vi "UHR-Fleezers Control (host) -TL FB Corrected Ronen semipassive.vi"(0 "Tab Control":T5(tab)=enum."Trap Control (RF)") -> ()   [LabVIEW 2013] (continued)
        n1854 = Array Subset(array=w2700, index (col)=w2689) -> (w2697:dbl[][])  [unwired: 3 in]
        n1855 = Array Subset(array=w2774, index (col)=0 ("index"), length (col)=w2689) -> (w2773:dbl[][])  [unwired: 2 in]
        n1856 = Array Subset(array=w2774, index (col)=w2689) -> (w2771:dbl[][])  [unwired: 3 in]
        n1857 = Array Subset(array=w2757, index (col)=0 ("index"), length (col)=w2689) -> (w2762:dbl[][])  [unwired: 2 in]
        n1858 = Array Subset(array=w2757, index (col)=w2689) -> (w2760:dbl[][])  [unwired: 3 in]
        n1859 = for {
          tunnel: w2769 -> [w2811] mode=indexing
          tunnel: [w2810] -> w2768 mode=indexing
          workers-P: _ -> [_]
          n1860 = Reverse 1D Array(array=w2811) -> (reversed array=w2810:dbl[])
        }
        n1861 = for {
          tunnel: w2755 -> [w2807] mode=indexing
          tunnel: [w2806] -> w2754 mode=indexing
          workers-P: _ -> [_]
          n1862 = Reverse 1D Array(array=w2807) -> (reversed array=w2806:dbl[])
        }
        n1863 = for {
          tunnel: w2699 -> [w2805] mode=indexing
          tunnel: [w2804] -> w2698 mode=indexing
          workers-P: _ -> [_]
          n1864 = Reverse 1D Array(array=w2805) -> (reversed array=w2804:dbl[])
        }
        n1865 = for {
          tunnel: w2773 -> [w2813] mode=indexing
          tunnel: [w2812] -> w2772 mode=indexing
          workers-P: _ -> [_]
          n1866 = Reverse 1D Array(array=w2813) -> (reversed array=w2812:dbl[])
        }
        n1867 = for {
          tunnel: w2762 -> [w2809] mode=indexing
          tunnel: [w2808] -> w2761 mode=indexing
          workers-P: _ -> [_]
          n1868 = Reverse 1D Array(array=w2809) -> (reversed array=w2808:dbl[])
        }
        n1869 = Index Array(array=w2774, index (row)=0) -> (element=→"Waveform Graph":dbl[])  [unwired: 1 in]
        n1870 = Add(x=w2768, y=w2767) -> (x+y=w2766:dbl[][])
        n1871 = Add(x=w2754, y=w2753) -> (x+y=w2752:dbl[][])
        n1872 = Add(x=w2698, y=w2697) -> (x+y=w2682:dbl[][])
        n1873 = Add(x=w2772, y=w2771) -> (x+y=w2746:dbl[][])
        n1874 = Add(x=w2761, y=w2760) -> (x+y=w2759:dbl[][])
        n1875 = Divide(x=w2752, y=2) -> (x/y=w2750:dbl[][])
        n1876 = Divide(x=w2766, y=2) -> (x/y=w2711:dbl[][])
        n1877 = Divide(x=w2759, y=2) -> (x/y=w2713:dbl[][])
        n1878 = To Single Precision Float(number=w2746) -> (single precision float=w2745:sgl[][])
        n1879 = Transpose 2D Array(2D array=w2750) -> (transposed array=→"Data map":dbl[][])
        n1880 = To Single Precision Float(number=w2682) -> (single precision float=w2686:sgl[][])
        n1881 = To Single Precision Float(number=w2711) -> (single precision float=w2717:sgl[][])
        n1882 = To Single Precision Float(number=w2713) -> (single precision float=w2714:sgl[][])
        n1883 = call "IMAQ ArrayToImage"("Image Pixels (Float)"=w2745, "Image"=w2679) -> ("Image Out"=w2748:T3)  [unwired: 8 in, 1 out]
        n1884 = call "IMAQ ArrayToImage"("Image Pixels (Float)"=w2686, "Image"=w2678) -> ("Image Out"=w2688:T3)  [unwired: 8 in, 1 out]
        n1885 = call "IMAQ ArrayToImage"("Image Pixels (Float)"=w2717, "Image"=w2677) -> ("Image Out"=w2719:T3)  [unwired: 8 in, 1 out]
        n1886 = call "IMAQ ArrayToImage"("Image Pixels (Float)"=w2714, "Image"=w2676) -> ("Image Out"=w2716:T3)  [unwired: 8 in, 1 out]
        n1887 = call "IMAQ Symmetry"("Type of Symmetry"=w2747, "Image Src"=w2748) -> ("Image Dst Out"=w2743:T3)  [unwired: 3 in, 1 out]
        n1888 = call "IMAQ Symmetry"("Type of Symmetry"=w2687, "Image Src"=w2688) -> ("Image Dst Out"=w2684:T3)  [unwired: 3 in, 1 out]
        n1889 = call "IMAQ Symmetry"("Type of Symmetry"=w2718, "Image Src"=w2719) -> ("Image Dst Out"=→"Detection Laser X":T3)  [unwired: 3 in, 1 out]
        n1890 = call "IMAQ Symmetry"("Type of Symmetry"=w2715, "Image Src"=w2716) -> ("Image Dst Out"=→"Detection Laser Y":T3)  [unwired: 3 in, 1 out]
        n1891 = call "IMAQ Set Simple Calibration"("Calibration Axis Info"=T37 {"Origin Pixel"={"X"=0.0, "Y"=0.0}, "Angle Relative to Horizontal (deg)"=0.0, "Axis Reference"=0}, "Grid Descriptor"=T38 {"X Step"=0.3, "Y Step"=0.3, "Unit"=enum."Undefined"}, "Image"=w2743) -> ("Calibrated Image"=→"APD 1":T3)  [unwired: 7 in, 1 out]
        n1892 = call "IMAQ Set Simple Calibration"("Calibration Axis Info"=T37 {"Origin Pixel"={"X"=0.0, "Y"=0.0}, "Angle Relative to Horizontal (deg)"=0.0, "Axis Reference"=0}, "Grid Descriptor"=T38 {"X Step"=0.3, "Y Step"=0.3, "Unit"=enum."Undefined"}, "Image"=w2684) -> ("Calibrated Image"=→"APD 2":T3)  [unwired: 7 in, 1 out]
      }
    }
    n1893 = Subtract(x=w2226, y="APD 2 Offset") -> (x-y=w2223:waveform(dbl))
    n1894 = Subtract(x=w2228, y="APD 1 Offset") -> (x-y=w2224:waveform(dbl))
    n1895 = Index Array(array=w2243, index=3) -> (element=w2310:waveform(dbl))
    n1896 = Index Array(array=w2243, index=6) -> (element=w2307:waveform(dbl))
    n1897 = Build Array(w2224, w2223) -> (→"APD Chart":waveform(dbl)[])
    n1898 = Array Size(array=w2300) -> (size(s)=w2350:i32)
    n1899 = call <vilib>:"Std Deviation and Variance.vi"("X"=w2236) -> ("standard deviation"=w2235:dbl)  [unwired: 1 in, 2 out]
    n1900 = Add Array Elements(numeric array=w2236) -> (sum=w2238:u32)
    n1901 = Add Array Elements(numeric array=w2300) -> (sum=w2360:u32)
    n1902 = call <vilib>:"Std Deviation and Variance.vi"("X"=w2300) -> ("standard deviation"=w2299:dbl)  [unwired: 1 in, 2 out]
    n1903 = Divide(x=w2235, y=w2234) -> (x/y=w2231:dbl)
    "Rate sigma (Hz) 2" <- w2231
    n1904 = Multiply(x=w2234, y=w2350) -> (x*y=w2237:dbl)
    "Int. Time (s)" <- w2237
    n1905 = Divide(x=w2238, y=w2237) -> (x/y=w2232:dbl)
    "APD 2 Rate (Hz)" <- w2232
    n1906 = Divide(x=w2360, y=w2237) -> (x/y=w2297:dbl)
    "APD 1 Rate (Hz)" <- w2297
    n1907 = Divide(x=w2299, y=w2234) -> (x/y=w2298:dbl)
    "Rate sigma (Hz)" <- w2298
    n1908 = Divide(x=w2231, y=w2232) -> (x/y=→"Sigma/Mean 2":dbl)
    n1909 = Divide(x=w2298, y=w2297) -> (x/y=→"Sigma/Mean":dbl)
    n1910 = case shown="2" "Calibration" {
      tunnel: "T1 alpha_x (nm/V)" -> [_ w2642 w2663]
      tunnel: "T1 kappa_x (pN/nm)" -> [_ _ w2653]
      tunnel: "T2 alpha_x (nm/V)" -> [_ w2641 w2661]
      tunnel: "T2 kappa_x (pN/nm)" -> [_ _ w2654]
      tunnel: w2310 -> [w2624 w2639 w2659]
      tunnel: w2307 -> [w2623 w2637 w2657]
      tunnel: [w2624 w2636 w2656] -> w2336
      tunnel: [w2623 w2635 w2655] -> w2335
      tunnel: ["T1 X (V)" ("Label.Text") "T1 X (nm)" ("Label.Text") "T1 X (pN)" ("Label.Text")] -> w2328
      tunnel: ["T2 X (V)" ("Label.Text") "T2 X (nm)" ("Label.Text") "T2 X (pN)" ("Label.Text")] -> w2327
      tunnel: ["Position (V)" ("Label.Text") "Position (nm)" ("Label.Text") "Force (pN)" ("Label.Text")] -> w2329
      tunnel: w2309 -> [_ w2627 w2646]
      tunnel: w2311 -> [_ w2630 w2648]
      tunnel: ["Mean (V)" ("Label.Text") "Mean (nm)" ("Label.Text") "Mean (pN)" ("Label.Text")] -> w2324
      tunnel: ["Difference (V)" ("Label.Text") "Difference (nm)" ("Label.Text") "Difference (pN)" ("Label.Text")] -> w2251
      frame 0, Default {
      }
      frame 1 {
        # "position"
        n1911 = Unbundle By Name(w2639) -> ("Y"=w2643:dbl[])
        n1912 = Unbundle By Name(w2637) -> ("Y"=w2628:dbl[])
        n1913 = Subtract(x=w2643, y=w2630) -> (x-y=w2631:dbl[])
        n1914 = Subtract(x=w2628, y=w2627) -> (x-y=w2629:dbl[])
        n1915 = Multiply(x=w2629, y=w2641) -> (x*y=w2638:dbl[])
        n1916 = Multiply(x=w2642, y=w2631) -> (x*y=w2640:dbl[])
        n1917 = Bundle By Name(cluster=w2637, "Y"=w2638) -> (w2635:waveform(dbl))
        n1918 = Bundle By Name(cluster=w2639, "Y"=w2640) -> (w2636:waveform(dbl))
      }
      frame 2 {
        # "force"
        n1919 = Unbundle By Name(w2659) -> ("Y"=w2664:dbl[])
        n1920 = Unbundle By Name(w2657) -> ("Y"=w2662:dbl[])
        n1921 = Subtract(x=w2662, y=w2646) -> (x-y=w2647:dbl[])
        n1922 = Subtract(x=w2664, y=w2648) -> (x-y=w2649:dbl[])
        n1923 = Compound Arithmetic op=MULTIPLY(w2647, w2661, w2654) -> (w2658:dbl[])
        n1924 = Compound Arithmetic op=MULTIPLY(w2653, w2663, w2649) -> (w2660:dbl[])
        n1925 = Bundle By Name(cluster=w2657, "Y"=w2658) -> (w2655:waveform(dbl))
        n1926 = Bundle By Name(cluster=w2659, "Y"=w2660) -> (w2656:waveform(dbl))
      }
    }
    n1927 = feedback-in #17("Calibration") -> ()
    n1928 = feedback #17(u16 1 ("Calibration")) -> (w2331:u16)
    n1929 = local read "Trap 2 Bead Size (nm)"() -> (w2131:dbl)
    n1930 = local read "Trap 1 Bead Size (nm)"() -> (w2130:dbl)
    n1931 = local read "AOM X Cal (nm/MHz)"() -> (w2128:dbl)
    n1932 = local read "Trap Delta (MHz)"() -> (w2127:dbl)
    n1933 = Not Equal?(x=w2331, y="Calibration") -> (x != y?=w2288:bool)
    n1934 = Multiply(x=w2128, y=w2127) -> (x*y=w2132:dbl)
    n1935 = Add(x=w2131, y=w2130) -> (x+y=w2134:dbl)
    n1936 = Unbundle By Name(w2310) -> ("Y"=w2313:dbl[])
    n1937 = Unbundle By Name(w2307) -> ("Y"=w2316:dbl[])
    n1938 = Divide(x=w2134, y=2.0) -> (x/y=w2129:dbl)
    n1939 = Subtract(x=w2313, y=w2311) -> (x-y=w2314:dbl[])
    n1940 = Subtract(x=w2316, y=w2309) -> (x-y=w2315:dbl[])
    n1941 = disable-structure shown="Enabled" {
      disable-tunnel: [-1.0 ("y") 1.0] -> w2317
      frame Disabled {
      }
      frame Enabled {
      }
    }
    n1942 = Multiply(x=w2315, y="T2 alpha_x (nm/V)") -> (x*y=w2306:dbl[])
    n1943 = Multiply(x="T1 alpha_x (nm/V)", y=w2314) -> (x*y=w2305:dbl[])
    n1944 = Multiply(x=w2335, y=w2317) -> (x*y=w2318:waveform(dbl))
    n1945 = case shown="False" "Read Lateness and Rel Phase" {
      tunnel: w2104 -> [w2590 w2612]
      tunnel: w2143 -> [w2591 w2611]
      tunnel: [w2590 w2610] -> w2303
      tunnel: [w2591 w2609] -> w2302
      frame False {
      }
      frame True {
        n1946 = xnode "Read/Write Control"("FPGA VI Reference In"=w2612, "error in"=w2611) -> ("FPGA VI Reference Out"=w2610:T20, "error out"=w2609:errorcluster, "GI Relative phase"=→"GI relative phase":i16, "Relative phase"=→"Relative phase (AI1)":i16, "AI Late Counter"=→"Late Counter (AI1)":u16, "GI Late Counter"=→"GI Late Counter":u16, "MCL Late Counter"=→"MCL Late Counter":u16, "MCL Relative Phase"=→"Relative Phase (MCL)":i16, "APD Acq Relative Phase"=→"APD Acq Relative Phase":i16, "APD 1 Gate Relative Phase"=→"APD 1 Gate Relative Phase":i16, "APD 2 Gate Relative Phase"=→"APD 2 Gate Relative Phase":i16, "APD Acq Late Counter"=→"APD Acq Late Counter":u16, "APD 1 Gate Late Counter"=→"APD 1 Gate Late Counter":u16, "APD 2 Gate Late Counter"=→"APD 2 Gate Late Counter":u16, "Green FB Relative Phase"=→"Relative phase (Green FB)":i16, "GI Relative phase 2"=→"GI relative phase 2":i16, "GI Late Counter 2"=→"GI Late Counter 2":u16, "Trap Pos FIFO Timeout"=→"Trap Pos FIFO Timeout":u16, "Trap AI FIFO Timeout"=→"Trap AI FIFO Timeout":u16)
      }
    }
    n1947 = Subtract(x=w2306, y=w2305) -> (x-y=w2126:dbl[])
    n1948 = call-poly <vilib>:"Mean.vi"("X"=w2126) -> ("mean"=w2133:dbl)  [unwired: 1 out]
    n1949 = Add(x=w2132, y=w2133) -> (x+y=w2136:dbl)
    n1950 = Subtract(x=w2136, y=w2129) -> (x-y=→"Tether Extension (nm, calculated)":dbl)
    n1951 = Unbundle By Name(w2335) -> ("Y"=w2276:dbl[])
    n1952 = Unbundle By Name(w2336) -> ("Y"=w2277:dbl[])
    n1953 = Build Array(w2336, w2318) -> (→"Force":waveform(dbl)[])
    n1954 = Subtract(x=w2126, y="Offset (nm)") -> (x-y=w2274:dbl[])
    n1955 = call-poly <vilib>:"Mean.vi"("X"=w2276) -> ("mean"=w2255:dbl)  [unwired: 1 out]
    "T2 X" <- w2255
    n1956 = Absolute Value(x=w2277) -> (abs(x)=w2278:dbl[])
    n1957 = Absolute Value(x=w2276) -> (abs(x)=w2279:dbl[])
    n1958 = call-poly <vilib>:"Mean.vi"("X"=w2277) -> ("mean"=w2256:dbl)  [unwired: 1 out]
    "T1 X" <- w2256
    n1959 = Add(x=w2278, y=w2279) -> (x+y=w2280:dbl[])
    n1960 = Bundle By Name(cluster=w2310, "Y"=w2274) -> (w2242:waveform(dbl))
    "Bead Separation" <- w2242
    n1961 = Divide(x=w2280, y=2.0) -> (x/y=→"Vec Mean of T1 T2":dbl[])
    n1962 = case shown="True" w2288 {
      tunnel: w2329 -> [_ w2617]
      tunnel: w2328 -> [_ w2616]
      tunnel: w2327 -> [_ w2615]
      tunnel: w2324 -> [_ w2614]
      tunnel: w2251 -> [_ w2613]
      frame False {
      }
      frame True {
        n1963 = property on="Force" class="WFChart (strict)"("YScale.NameLbl.Text"=w2617) -> ()  [unwired: 2 in, 2 out]
        n1964 = property on="T2 X" class="DigNum (strict)"("Caption.Text"=w2615) -> ()  [unwired: 2 in, 2 out]
        n1965 = property on="T1 X" class="DigNum (strict)"("Caption.Text"=w2616) -> ()  [unwired: 2 in, 2 out]
        n1966 = property on="Mean" class="DigNum (strict)"("Caption.Text"=w2614) -> ()  [unwired: 2 in, 2 out]
        n1967 = property on="Difference" class="DigNum (strict)"("Caption.Text"=w2613) -> ()  [unwired: 2 in, 2 out]
      }
    }
    n1968 = local read "Tether"() -> (w2282:bool)
    n1969 = Absolute Value(x=w2256) -> (abs(x)=w2253:dbl)
    n1970 = Absolute Value(x=w2255) -> (abs(x)=w2252:dbl)
    n1971 = Add(x=w2253, y=w2252) -> (x+y=w2326:dbl)
    n1972 = Subtract(x=w2253, y=w2252) -> (x-y=→"Difference":dbl)
    n1973 = feedback #18(w2274) -> (w2273:dbl[])
    n1974 = Divide(x=w2326, y=2.0) -> (x/y=w2101:dbl)
    "Mean" <- w2101
    n1975 = case shown="True" w2282 {
      tunnel: w2101 -> [_ w2549]
      frame False {
      }
      frame True {
        n1976 = Greater?(x="Lost Tether Alarm Threshold (pN)", y=w2549) -> (0:w2547:bool)
        n1977 = case shown="True" w2547 {
          frame False {
          }
          frame True {
            n1978 = flat-sequence {
              frame #0 {
                # "stop only if saving"
                n1979 = local read "Saving..."() -> (w2562:bool)
                n1980 = And(x=w2562, y="TA Cancel Save?") -> (x .and. y?=w2561:bool)
                n1981 = local write "Stop Saving"(w2561) -> ()
              }
              frame #1 {
                n1982 = case shown="True" "TA Green Off?" {
                  frame False {
                  }
                  frame True {
                    w2565 = FALSE ("Fl. Triggered...")
                    n1983 = local write "Fl. Triggered..."(w2565) -> ()
                    n1984 = property on="Green Laser ON/Interlacing" class="Bool (strict)"("Val(Sgnl)"=w2565) -> ()  [unwired: 2 in, 2 out]
                  }
                }
              }
            }
            n1985 = local read "Time tether formed"() -> (w2556:timestamp)
            n1986 = Get Date/Time In Seconds() -> (seconds since 1Jan1904=w2557:timestamp)
            n1987 = Subtract(x=w2557, y=w2556) -> (x-y=w2555:dbl)
            n1988 = Number To Decimal String(number=w2555) -> (decimal integer string=w2552:string)  [unwired: 1 out]
            n1989 = local read "Messages"() -> (w2559:string)
            n1990 = call <vilib>:"Beep.vi"() -> ()  [unwired: 3 in, 9 out]
            n1991 = Concatenate Strings("Lost tether (" ("Message to add"), w2552, " s)." ("string")) -> (w2554:string)
            n1992 = local write "Tether"(FALSE ("Tether")) -> ()
            n1993 = call "Update messages.vi"("Message to add"=w2554, "Old message string"=w2559) -> ("New message string"=w2558:string)
            n1994 = local write "Messages"(w2558) -> ()
            n1995 = property on="Trap Pos. FB ON" class="Bool (strict)"("Val(Sgnl)"=FALSE ("Value (Signaling)")) -> ()  [unwired: 2 in, 2 out]
          }
        }
      }
    }
    n1996 = Build Array (concatenate)(w2274, w2273) -> (w2272:dbl[])
    n1997 = Split 1D Array(array=w2272, index=w2154) -> (first subarray=w2268:dbl[])  [unwired: 1 out]
    n1998 = feedback-in #18(w2268) -> ()
    n1999 = call-poly <vilib>:"Mean.vi"("X"=w2268) -> ("mean"=w2267:dbl)  [unwired: 1 out]
    "Bead Mean (nm)" <- w2267
    n2000 = Subtract(x=w2268, y=w2267) -> (x-y=w2266:dbl[])
    n2001 = Square(x=w2266) -> (x^2=w2265:dbl[])
    n2002 = case shown="True" "Semi Passive ON" {
      tunnel: "Semi Passive mode" -> [_ w2428]
      tunnel: "Jump Force (pN)" -> [_ w2427]
      tunnel: w2101 -> [_ w2426]
      frame False {
      }
      frame True {
        n2003 = case shown="\"Use Feedback\"" w2428 {
          tunnel: w2427 -> [_ w2431 w2447]
          tunnel: w2426 -> [_ w2430 w2446]
          frame "None" {
          }
          frame "Use Feedback" {
            n2004 = local read "Target Force (pN)"() -> (w2433:dbl)
            n2005 = Less?(x=w2431, y=w2433) -> (x < y?=w2432:bool)
            n2006 = case shown="True" w2432 {
              tunnel: w2431 -> [w2440 w2443]
              tunnel: w2430 -> [w2439 w2442]
              tunnel: [w2438 w2441] -> w2429
              frame False {
                n2007 = Less?(x=w2440, y=w2439) -> (x < y?=w2438:bool)
              }
              frame True {
                n2008 = Greater?(x=w2443, y=w2442) -> (0:w2441:bool)
              }
            }
            n2009 = case shown="True" w2429 {
              frame False {
                n2010 = local read "Trap Pos. FB ON"() -> (w2434:bool)
                n2011 = case shown="True" w2434 {
                  frame False {
                  }
                  frame True {
                    n2012 = property on="Trap Pos. FB ON" class="Bool (strict)"("Val(Sgnl)"=FALSE) -> ()  [unwired: 2 in, 2 out]
                  }
                }
              }
              frame True {
                n2013 = local read "Trap Pos. FB ON"() -> (w2436:bool)
                n2014 = case shown="False" w2436 {
                  frame False {
                    n2015 = property on="Trap Pos. FB ON" class="Bool (strict)"("Val(Sgnl)"=TRUE) -> ()  [unwired: 2 in, 2 out]
                  }
                  frame True {
                  }
                }
              }
            }
          }
          frame "Sharp Jump" {
            n2016 = local read "Target Force (pN)"() -> (w2449:dbl)
            n2017 = Greater?(x=w2447, y=w2449) -> (0:w2448:bool)
            n2018 = case shown="True" w2448 {
              tunnel: w2447 -> [w2464 w2468]
              tunnel: w2446 -> [w2465 w2467]
              tunnel: [w2463 w2466] -> w2445
              frame False {
                n2019 = Greater?(x=w2465, y=w2464) -> (0:w2463:bool)
              }
              frame True {
                n2020 = Less?(x=w2468, y=w2467) -> (x < y?=w2466:bool)
              }
            }
            n2021 = Subtract(x=w2447, y=w2449) -> (x-y=w2444:dbl)
            n2022 = case shown="True" w2445 {
              tunnel: w2444 -> [_ w2455]
              frame False {
              }
              frame True {
                n2023 = local read "T1 kappa_x (pN/nm)"() -> (w2460:dbl)
                n2024 = local read "T2 kappa_x (pN/nm)"() -> (w2461:dbl)
                n2025 = Reciprocal(x="DNA stiffness (pN / nm)") -> (1/x=w2457:dbl)
                n2026 = Reciprocal(x=w2460) -> (1/x=w2459:dbl)
                n2027 = Reciprocal(x=w2461) -> (1/x=w2458:dbl)
                n2028 = Compound Arithmetic op=ADD(w2459, w2458, w2457) -> (w2456:dbl)
                n2029 = local read "AOM X Cal (nm/MHz)"() -> (w2454:dbl)
                n2030 = Multiply(x=w2456, y=w2455) -> (x*y=w2453:dbl)
                n2031 = local read "Trap Delta (MHz)"() -> (w2451:dbl)
                n2032 = Divide(x=w2453, y=w2454) -> (x/y=w2452:dbl)
                n2033 = Subtract(x=w2451, y=w2452) -> (x-y=w2450:dbl)
                n2034 = property on="Trap Delta (MHz)" class="DigNum (strict)"("Val(Sgnl)"=w2450) -> ()  [unwired: 2 in, 2 out]
              }
            }
          }
        }
      }
    }
    n2035 = call-poly <vilib>:"Mean.vi"("X"=w2265) -> ("mean"=w2264:dbl)  [unwired: 1 out]
    n2036 = Square Root(x=w2264) -> (sqrt(x)=w2263:dbl)
    n2037 = Multiply(x=10.0, y=w2263) -> (x*y=→"RMS (Ang)":dbl)
    n2038 = xnode "Read/Write Control"("FPGA VI Reference In"=w2303, "error in"=w2302) -> ("FPGA VI Reference Out"=w2414:T20, "error out"=w2408:errorcluster, "AI4 Y Sum Set 1"=w2404:i16, "AI4 Y Sum Set 2"=w2403:i16, "AI1 X Set 1"=w2188:fxp<+/-,16,1>, "AI1 X Set 2"=w2187:fxp<+/-,16,1>, "Trap Pos FB Int Signal"=→"Trap Pos FB Int Signal":fxp<+/-,24,9>, "Trap Pos FB Int-Norm Signal"=→"Trap Pos FB Int-Norm Signal":fxp<+/-,24,9>, "Trap Pos FB Action"=w2181:i64, "Scanning"=→"AOD Scanning":bool, "Scan I"=→"AOD Scan I":u64, "Scanning MCL"=w2406:bool, "Scan I (MCL)"=→"MCL Scan I":u64, "Green FB Signals"=w2345:T48)  [unwired: 1 out]
    "MCL Scanning" <- w2406
    "Trap Pos FB Action" <- w2181
    n2039 = local read "AI2 (V)"() -> (w2405:cluster{"Set 1":dbl, "Set 2":dbl})
    n2040 = Bundle By Name(cluster=w2405, "Set 1"=w2404, "Set 2"=w2403) -> (w2401:cluster{"Set 1":dbl, "Set 2":dbl})
    n2041 = Divide(x=w2181, y=327.67) -> (x/y=→"Action (%)":dbl)
    n2042 = local read "Trap X (AI1)"() -> (w2201:T1)
    n2043 = Divide(x=w2401, y=3276.7) -> (x/y=w2400:cluster{"Set 1":dbl, "Set 2":dbl})
    n2044 = local write "AI2 (V)"(w2400) -> ()
    n2045 = Bundle(cluster=w2201, "Trap 1"=w2188, "Trap 2"=w2187) -> (→"Trap X (AI1)":T1)
    n2046 = Divide(x=w2345, y=3276.7) -> (x/y=w2341:T49)
    n2047 = Unbundle By Name(w2341) -> ("Green FB Ch 0"=w2344:dbl, "Green FB Ch 1"=w2343:dbl, "Green FB Ch 2"=w2342:dbl)
    n2048 = Divide(x=w2344, y=w2342) -> (x/y=w2340:dbl)
    n2049 = Divide(x=w2343, y=w2342) -> (x/y=w2339:dbl)
    n2050 = flat-sequence "To save data" {
      tunnel: [w3439] -> w2425
      tunnel: [w3440] -> w2424
      tunnel: w2376 -> [w3433]
      tunnel: w2270 -> [w3437]
      tunnel: ["Save Calibration"] -> w2397
      tunnel: w2394 -> [w3436]
      tunnel: [w3429] -> w2393
      tunnel: [w3426] -> w2392
      tunnel: [w3423] -> w2391
      tunnel: w2375 -> [w3425]
      tunnel: w2286 -> [w3419]
      tunnel: [w3419] -> w2285
      tunnel: ["Start Saving"] -> w2244
      tunnel: [w3413] -> w2170
      tunnel: [w3412] -> w2169
      tunnel: w2425 -> [w3674]
      tunnel: w2424 -> [w3673]
      tunnel: w2171 -> [w3672]
      tunnel: w2397 -> [w3671]
      tunnel: w2393 -> [w3669]
      tunnel: w2392 -> [w3668]
      tunnel: w2391 -> [w3667]
      tunnel: w2257 -> [w3666]
      tunnel: w2295 -> [w3665]
      tunnel: w2285 -> [w3664]
      tunnel: w2244 -> [w3663]
      tunnel: w2242 -> [w3662]
      tunnel: w2218 -> [w3661]
      tunnel: w2170 -> [w3660]
      tunnel: w2169 -> [w3659]
      tunnel: w2168 -> [w3658]
      frame #0 {
        n2051 = Or(x="Save N Sets", y="Start Saving") -> (x .or. y?=w3420:bool)
        n2052 = To Double Precision Float(number=w3436) -> (double precision float=w3430:dbl)
        n2053 = Build Array(w3420, "Save Calibration", w3433, w3425) -> (w3435:bool[])
        n2054 = Compound Arithmetic op=OR("Save Calibration", w3433, w3420, w3425) -> (w3438:bool)
        n2055 = Boolean Array To Number(Boolean array=w3435) -> (number=w3432:u32)
        n2056 = feedback #19(FALSE ("Save APD Data\nwith Trap Data")) -> (w3414:bool)
        n2057 = feedback #20(refnum<k0> refnum) -> (w3441:refnum<file>)
        n2058 = feedback #21(refnum<k0> refnum) -> (w3416:refnum<file>)
        n2059 = feedback #22(FALSE ("Save APD Data\nwith Trap Data")) -> (w3424:bool)
        n2060 = feedback #23(refnum<k0> refnum) -> (w3427:refnum<file>)
        n2061 = feedback #24(0) -> (w3443:i32)
        n2062 = feedback #25() -> (w3431:u32)  [unwired: 1 out]
        n2063 = case shown="True" w3438 {
          tunnel: [w3450 1] -> w3439
          tunnel: w3443 -> [w3452 _]
          tunnel: [w3451 w3470] -> w3440
          tunnel: w3441 -> [w3451 _]
          tunnel: w3437 -> [_ w3490]
          tunnel: w3430 -> [_ w3488]
          tunnel: w3432 -> [_ w3491]
          tunnel: [w3449 w3469] -> w3429
          tunnel: w3431 -> [w3449 _]
          tunnel: [w3448 w3467] -> w3426
          tunnel: w3427 -> [w3448 _]
          tunnel: [w3447 w3466] -> w3423
          tunnel: w3424 -> [w3447 _]
          tunnel: "Start Saving" -> [_ w3464]
          tunnel: w3419 -> [_ w3463]
          tunnel: [w3446 w3454] -> w3412
          tunnel: w3416 -> [w3446 _]
          tunnel: [w3445 w3453] -> w3413
          tunnel: w3414 -> [w3445 _]
          frame False {
            n2064 = Increment(x=w3452) -> (x+1=w3450:i32)
          }
          frame True {
            w3460 = FALSE ("Start Saving")
            w3465 = 9.0  # File Version
            w3473 = FALSE ("prepend array or string size? (T)")
            w3471 = T30."big-endian, network order" ("byte order (0:big-endian, network order)")
            # "write file headers"
            n2065 = local read "BD 1 Frequency 1 (MHz)"() -> (w3487:dbl)
            n2066 = local read "BD 2 Frequency 1 (MHz)"() -> (w3486:dbl)
            n2067 = local read "BD 1 Frequency 2 (MHz)"() -> (w3485:dbl)
            n2068 = local read "BD 2 Frequency 2 (MHz)"() -> (w3484:dbl)
            n2069 = local read "BD 1 Frequency 3 (MHz)"() -> (w3483:dbl)
            n2070 = local read "BD 2 Frequency 3 (MHz)"() -> (w3482:dbl)
            n2071 = Array Size(array=w3463) -> (size(s)=w3462:i32)
            n2072 = To Double Precision Float(number=w3462) -> (double precision float=w3461:dbl)
            n2073 = local write "Save Calibration"(w3460) -> ()
            n2074 = local write "Start Saving"(w3460) -> ()
            n2075 = Build Array("Save APD Data\nwith Trap Data", "Save Trap Pos. Data") -> (w3457:bool[])
            n2076 = Boolean Array To Number(Boolean array=w3457) -> (number=w3456:u32)
            n2077 = Build Array(w3487, w3486, w3485, w3484, w3483, w3482) -> (w3481:dbl[])
            n2078 = case shown="4" w3491 {
              tunnel: w3490 -> [w3562 w3582 w3598 w3636]
              tunnel: w3461 -> [w3567 w3589 w3618 w3655]
              tunnel: w3488 -> [w3566 w3588 w3617 w3654]
              tunnel: [w3563 w3584 w3609 w3646] -> w3479
              tunnel: [w3554 "Cal sets to save" w3599 w3637] -> w3469
              tunnel: w3481 -> [w3564 w3585 w3611 w3648]
              tunnel: "Save APD Data\nwith Trap Data" -> [w3561 _ w3595 w3634]
              tunnel: [w3561 w3576 w3595 w3634] -> w3466
              tunnel: w3465 -> [w3557 w3577 w3593 w3632]
              tunnel: w3464 -> [w3556 _ _ _]
              tunnel: [w3547 w3576 w3592 w3622] -> w3453
              tunnel: "Save Trap Pos. Data" -> [w3547 _ w3592 w3622]
              tunnel: w3456 -> [w3546 _ w3591 w3621]
              frame 1, Default {
                # "timeseries"
                n2079 = case shown="True" "Profile" {
                  tunnel: [w3570 w3573] -> w3551
                  tunnel: [w3570 w3572] -> w3550
                  tunnel: [w3570 w3571] -> w3549
                  tunnel: [w3570 w3575] -> w3548
                  frame False {
                    w3570 = 0.0 ("f")
                  }
                  frame True {
                    n2080 = local read "Current Position"() -> (w3574:dbl[])
                    n2081 = local read "Y change (mm)"() -> (w3575:dbl)
                    n2082 = call "subVI_explode3array.vi"("Array"=w3574) -> ("x"=w3573:dbl, "y"=w3572:dbl, "z"=w3571:dbl)  [unwired: 12 in]
                  }
                }
                n2083 = local read "Save ave N"() -> (w3569:dbl)
                n2084 = Multiply(x=w3569, y=w3562) -> (x*y=w3568:dbl)
                n2085 = To Double Precision Float(number=w3546) -> (double precision float=w3560:dbl)
                n2086 = Build Array(w3557, w3562, w3568, w3567, w3566, 0.0 ("f")) -> (w3565:dbl[])
                n2087 = Build Array(w3560, w3551, w3550, w3549, w3548) -> (w3558:dbl[])
                n2088 = Select(t=u32 4000000000, s=w3556, f="N sets to save") -> (s? t:f=w3554:u32)
                n2089 = Build Array (concatenate)(w3565, w3564, w3558) -> (w3563:dbl[])
              }
              frame 2 {
                w3579 = 0.0 ("f")
                w3576 = FALSE ("Save APD Data\nwith Trap Data")
                # "calibration"
                n2090 = Boolean To (0,1)(Boolean=w3576) -> (0, 1=w3581:i16)
                n2091 = To Double Precision Float(number=w3581) -> (double precision float=w3580:dbl)
                n2092 = Build Array(w3580, w3579, w3579, w3579, w3579) -> (w3578:dbl[])
                n2093 = Build Array(w3577, w3582, w3582, w3589, w3588, 1.0 ("t")) -> (w3586:dbl[])
                n2094 = Build Array (concatenate)(w3586, w3585, w3578) -> (w3584:dbl[])
                "Calibrating Trap..." <- TRUE ("Calibrating...")
              }
              frame 4 {
                w3596 = 0.0 ("f")
                # "write file header for a trap \nraster scan"
                # "scan dir (x/y = 0/1)"
                # "cycles/step"
                # "n scans (f/b)"
                # "steps"
                # "freq. range"
                # "AOD raster scan"
                n2095 = local read "Number of F/B Scans (AOD)"() -> (w3603:u16)
                n2096 = local read "Cycles/step (AOD)"() -> (w3605:u64)
                n2097 = local read "Scan Range (MHz)"() -> (w3608:dbl)
                n2098 = local read "Scan steps (AOD)"() -> (w3607:u64)
                n2099 = local read "Scan BD"() -> (w3615:bool)
                n2100 = local read "Save ave N"() -> (w3620:dbl)
                n2101 = Boolean To (0,1)(Boolean=w3615) -> (0, 1=w3614:i16)
                n2102 = To Double Precision Float(number=w3603) -> (double precision float=w3602:dbl)
                n2103 = To Double Precision Float(number=w3607) -> (double precision float=w3606:dbl)
                n2104 = To Double Precision Float(number=w3605) -> (double precision float=w3604:dbl)
                n2105 = To Double Precision Float(number=w3614) -> (double precision float=w3613:dbl)
                n2106 = Multiply(x=w3620, y=w3598) -> (x*y=w3619:dbl)
                n2107 = To Double Precision Float(number=w3591) -> (double precision float=w3597:dbl)
                n2108 = Build Array(w3597, w3596, w3596, w3596, w3596) -> (w3594:dbl[])
                n2109 = local read "N sets should be saved"() -> (w3600:dbl)
                n2110 = Build Array(w3613, w3608, w3606, w3604, w3602) -> (w3610:dbl[])
                n2111 = Build Array(w3593, w3598, w3619, w3618, w3617, 2.0 ("t")) -> (w3612:dbl[])
                n2112 = Round Toward +Infinity(x=w3600) -> (ceil(x): smallest int >= x=w3601:dbl)
                n2113 = Build Array (concatenate)(w3612, w3611, w3594, w3610) -> (w3609:dbl[])
                n2114 = To Unsigned Long Integer(number=w3601) -> (unsigned 32bit integer=w3599:u32)
              }
              frame 8 {
                w3629 = 0.0 ("f")
                # "MCL raster scan"
                n2115 = local read "Number of scans (MCL)"() -> (w3624:u64)
                n2116 = local read "Scan lines (y)"() -> (w3623:u64)
                n2117 = local read "2D or 1D Scan"() -> (w3626:bool)
                n2118 = local read "Scan Range (V)\n(of steps)"() -> (w3645:dbl)
                n2119 = local read "Fast Scan Dir"() -> (w3652:bool)
                n2120 = local read "Cycles/step (MCL)"() -> (w3642:u64)
                n2121 = local read "Scan steps (MCL)"() -> (w3644:u64)
                n2122 = Select(t=w3623, s=w3626, f=w3624) -> (s? t:f=w3625:u64)
                n2123 = Boolean To (0,1)(Boolean=w3626) -> (0, 1=w3628:i16)
                n2124 = local read "Save ave N"() -> (w3657:dbl)
                n2125 = local read "Initial X"() -> (w3631:dbl)
                n2126 = local read "Initial Y"() -> (w3630:dbl)
                n2127 = To Double Precision Float(number=w3628) -> (double precision float=w3627:dbl)
                n2128 = Boolean To (0,1)(Boolean=w3652) -> (0, 1=w3651:i16)
                n2129 = To Double Precision Float(number=w3625) -> (double precision float=w3640:dbl)
                n2130 = To Double Precision Float(number=w3644) -> (double precision float=w3643:dbl)
                n2131 = To Double Precision Float(number=w3642) -> (double precision float=w3641:dbl)
                n2132 = To Double Precision Float(number=w3651) -> (double precision float=w3650:dbl)
                n2133 = Multiply(x=w3657, y=w3636) -> (x*y=w3656:dbl)
                n2134 = To Double Precision Float(number=w3621) -> (double precision float=w3635:dbl)
                n2135 = local read "N sets should be saved (MCL)"() -> (w3638:dbl)
                n2136 = Build Array(w3635, w3627, w3629, w3629, w3629) -> (w3633:dbl[])
                n2137 = Build Array(w3650, w3645, w3643, w3641, w3640, w3631, w3630) -> (w3647:dbl[])
                n2138 = Build Array(w3632, w3636, w3656, w3655, w3654, 3.0 ("t")) -> (w3649:dbl[])
                n2139 = Round Toward +Infinity(x=w3638) -> (ceil(x): smallest int >= x=w3639:dbl)
                n2140 = Build Array (concatenate)(w3649, w3648, w3633, w3647) -> (w3646:dbl[])
                n2141 = To Unsigned Long Integer(number=w3639) -> (unsigned 32bit integer=w3637:u32)
              }
            }
            n2142 = local read "Index"() -> (w3496:dbl)
            n2143 = call "Create new save file.vi"("Insert"="", "Ext"=".dat", "Index In"=w3496) -> ("Path Out"=w3455:path, "Index Out"=w3468:dbl)
            n2144 = local write "Save file name"(w3455) -> ()
            n2145 = local write "Index"(w3468) -> ()
            n2146 = local write "Save index"(w3468) -> ()
            n2147 = Array Size(array=w3479) -> (size(s)=w3480:i32)
            n2148 = Open/Create/Replace File(file path (use dialog)=w3455, operation (0:open)=T24."create", access (0:read/write)=enum16{"read/write", "read-only", "write-only"}."write-only") -> (refnum out=w3493:refnum<file>)  [unwired: 1 in, 4 out]
            n2149 = local write "Saving..."(TRUE ("Saving...")) -> ()
            n2150 = To Double Precision Float(number=w3480) -> (double precision float=w3478:dbl)
            n2151 = String Length(string="Comment (data description)") -> (length=w3476:i32)
            n2152 = To Double Precision Float(number=w3476) -> (double precision float=w3475:dbl)
            n2153 = Deny Access(7:w3493) -> (3:w3492:refnum<file>)  [unwired: 1 in, 2 out]
            n2154 = Build Array (concatenate)(w3478, w3479, w3475) -> (w3477:dbl[])
            n2155 = case "If fluorescence data to be saved" shown="True" w3466 {
              tunnel: w3455 -> [_ w3545]
              tunnel: [refnum<k0> refnum w3525] -> w3467
              frame False {
              }
              frame True {
                w3524 = 0.0
                n2156 = local read "APD Integration Time (s)"() -> (w3530:dbl)
                n2157 = local read "N APD Samp/step"() -> (w3523:dbl)
                n2158 = Path To String(path=w3545) -> (string=w3544:string)
                n2159 = String Length(string=w3544) -> (length=w3543:i32)
                n2160 = Subtract(x=w3543, y=4) -> (x-y=w3541:i32)
                n2161 = String Subset(string=w3544, length (rest)=w3541) -> (substring=w3540:string)  [unwired: 1 out]
                n2162 = Build Array(w3530, w3523, w3524, w3524, w3524, w3524, w3524, w3524) -> (w3527:dbl[])
                n2163 = Concatenate Strings(w3540, "_fl.dat" ("string")) -> (w3538:string)
                n2164 = Array Size(array=w3527) -> (size(s)=w3529:i32)
                n2165 = String To Path(string=w3538) -> (path=w3534:path)
                n2166 = Open/Create/Replace File(file path (use dialog)=w3534, operation (0:open)=T24."create", access (0:read/write)=enum16{"read/write", "read-only", "write-only"}."write-only") -> (refnum out=w3535:refnum<file>)  [unwired: 1 in, 4 out]
                n2167 = Deny Access(7:w3535) -> (3:w3531:refnum<file>)  [unwired: 1 in, 2 out]
                n2168 = To Double Precision Float(number=w3529) -> (double precision float=w3528:dbl)
                n2169 = Build Array (concatenate)(w3528, w3527) -> (w3526:dbl[])
                n2170 = Write to Binary File(file (use dialog)=w3531, data=w3526, 5:FALSE ("prepend array or string size? (T)"), 9:T30."big-endian, network order" ("byte order (0:big-endian, network order)")) -> (refnum out=w3525:refnum<file>)  [unwired: 1 in, 3 out]
              }
            }
            n2171 = case shown="True" w3453 {
              tunnel: w3455 -> [_ w3507]
              tunnel: [refnum<k0> refnum w3506] -> w3454
              frame False {
              }
              frame True {
                w3502 = 0.0 ("element")
                n2172 = Path To String(path=w3507) -> (string=w3521:string)
                n2173 = Build Array(w3502, w3502, w3502, w3502, w3502, w3502, w3502, w3502) -> (w3503:dbl[])
                n2174 = String Length(string=w3521) -> (length=w3520:i32)
                n2175 = Subtract(x=w3520, y=4) -> (x-y=w3518:i32)
                n2176 = Array Size(array=w3503) -> (size(s)=w3505:i32)
                n2177 = String Subset(string=w3521, length (rest)=w3518) -> (substring=w3517:string)  [unwired: 1 out]
                n2178 = To Double Precision Float(number=w3505) -> (double precision float=w3504:dbl)
                n2179 = Concatenate Strings(w3517, "_pos.dat" ("string")) -> (w3515:string)
                n2180 = Build Array (concatenate)(w3504, w3503) -> (w3501:dbl[])
                n2181 = String To Path(string=w3515) -> (path=w3511:path)
                n2182 = Open/Create/Replace File(file path (use dialog)=w3511, operation (0:open)=T24."create", access (0:read/write)=enum16{"read/write", "read-only", "write-only"}."write-only") -> (refnum out=w3512:refnum<file>)  [unwired: 1 in, 4 out]
                n2183 = Deny Access(7:w3512) -> (3:w3508:refnum<file>)  [unwired: 1 in, 2 out]
                n2184 = Write to Binary File(file (use dialog)=w3508, data=w3501, 5:FALSE ("prepend array or string size? (T)"), 9:T30."big-endian, network order" ("byte order (0:big-endian, network order)")) -> (refnum out=w3506:refnum<file>)  [unwired: 1 in, 3 out]
              }
            }
            n2185 = Write to Binary File(file (use dialog)=w3492, data=w3477, 5:w3473, 9:w3471) -> (refnum out=w3474:refnum<file>)  [unwired: 1 in, 3 out]
            n2186 = Write to Binary File(file (use dialog)=w3474, data="Comment (data description)", 5:w3473, 9:w3471) -> (refnum out=w3470:refnum<file>)  [unwired: 1 in, 3 out]
          }
        }
        n2187 = feedback-in #19(w3413) -> ()
        n2188 = feedback-in #20(w3440) -> ()
        n2189 = feedback-in #21(w3412) -> ()
        n2190 = feedback-in #22(w3423) -> ()
        n2191 = feedback-in #23(w3426) -> ()
        n2192 = feedback-in #24(w3439) -> ()
        n2193 = feedback-in #25(w3429) -> ()
      }
      frame #1 {
        n2194 = local read "Saving..."() -> (w3670:bool)
        n2195 = case shown="True" w3670 {
          tunnel: w3674 -> [_ w3684]
          tunnel: w3673 -> [_ w3698]
          tunnel: w3672 -> [_ w3694]
          tunnel: w3671 -> [_ w3693]
          tunnel: w3669 -> [_ w3692]
          tunnel: w3668 -> [_ w3687]
          tunnel: w3667 -> [_ w3686]
          tunnel: w3666 -> [_ w3685]
          tunnel: w3665 -> [_ w3683]
          tunnel: w3664 -> [_ w3681]
          tunnel: w3663 -> [_ w3680]
          tunnel: w3662 -> [_ w3679]
          tunnel: w3661 -> [_ w3678]
          tunnel: w3660 -> [_ w3677]
          tunnel: w3659 -> [_ w3676]
          tunnel: w3658 -> [_ w3675]
          frame False {
          }
          frame True {
            n2196 = Multiply(x=w3684, y=w3683) -> (x*y=→"Time (s)":dbl)
            n2197 = Less Or Equal?(x=w3684, y=w3692) -> (x <= y?=w3696:bool)
            n2198 = Or(x="Stop Saving", y="Abort save 2") -> (x .or. y?=w3688:bool)
            n2199 = Not(x=w3688) -> (.not. x?=w3697:bool)
            n2200 = And(x=w3696, y=w3697) -> (x .and. y?=w3695:bool)
            n2201 = case shown="True" w3695 {
              tunnel: w3698 -> [w3705 w3773]
              tunnel: [0.0 w3776] -> w3691
              tunnel: w3684 -> [_ w3774]
              tunnel: w3692 -> [_ w3775]
              tunnel: w3694 -> [_ w3770]
              tunnel: w3693 -> [_ _]
              tunnel: w3687 -> [w3703 w3763]
              tunnel: w3686 -> [w3702 w3764]
              tunnel: w3685 -> [_ w3762]
              tunnel: w3681 -> [_ w3761]
              tunnel: w3680 -> [_ w3715]
              tunnel: w3679 -> [_ w3754]
              tunnel: w3678 -> [_ w3732]
              tunnel: w3677 -> [w3700 w3713]
              tunnel: w3676 -> [w3701 w3712]
              tunnel: w3675 -> [_ w3709]
              frame False {
                w3699 = FALSE
                n2202 = Close File(refnum=w3705) -> ()  [unwired: 1 in, 2 out]
                n2203 = case shown="True" w3702 {
                  tunnel: w3703 -> [_ w3707]
                  frame False {
                  }
                  frame True {
                    n2204 = Close File(refnum=w3707) -> ()  [unwired: 1 in, 2 out]
                  }
                }
                n2205 = case shown="True" w3700 {
                  tunnel: w3701 -> [_ w3706]
                  frame False {
                  }
                  frame True {
                    n2206 = Close File(refnum=w3706) -> ()  [unwired: 1 in, 2 out]
                  }
                }
                n2207 = local write "Calibrating Trap..."(w3699) -> ()
                n2208 = call <vilib>:"Beep.vi"() -> ()  [unwired: 3 in, 9 out]
                n2209 = local write "Stop Saving"(w3699) -> ()
                n2210 = property on="Raster Scanning..." class="Bool (strict)"("Val(Sgnl)"=w3699) -> ()  [unwired: 2 in, 2 out]
                "Saving..." <- w3699
              }
              frame True {
                n2211 = local read "Calibrating Trap..."() -> (w3765:bool)
                n2212 = case "Write fl. data" shown="True" w3764 {
                  tunnel: w3763 -> [_ w3799]
                  tunnel: w3762 -> [_ w3798]
                  frame False {
                  }
                  frame True {
                    n2213 = Write to Binary File(file (use dialog)=w3799, data=w3798, 5:FALSE ("prepend array or string size? (T)"), 9:T30."big-endian, network order" ("byte order (0:big-endian, network order)")) -> ()  [unwired: 1 in, 4 out]
                  }
                }
                n2214 = Greater?(x="Save ave N", y=1.0) -> (0:w3768:bool)
                n2215 = Not(x=w3765) -> (.not. x?=w3767:bool)
                n2216 = And(x=w3767, y=w3768) -> (x .and. y?=w3710:bool)
                n2217 = case shown="True" w3710 {
                  tunnel: w3709 -> [w3779 w3790]
                  tunnel: [w3779 w3782] -> w3708
                  tunnel: "Save ave N" -> [_ w3783]
                  frame False {
                  }
                  frame True {
                    w3780 = 2 ("dimension size")
                    n2218 = Array Size(array=w3790) -> (size(s)=w3784:i32)
                    n2219 = Divide(x=w3784, y=w3780) -> (x/y=w3788:dbl)
                    n2220 = Reshape Array(w3790, w3788, w3780) -> (w3789:u64[][])
                    n2221 = Transpose 2D Array(2D array=w3789) -> (transposed array=w3787:u64[][])
                    n2222 = for {
                      tunnel: w3787 -> [w3792] mode=indexing
                      tunnel: [w3791] -> w3781 mode=indexing
                      tunnel: w3783 -> [w3793]
                      workers-P: _ -> [_]
                      n2223 = call "downsample 1D array - U64.vi"("Ave N"=w3793, "Array In"=w3792) -> ("Array Out"=w3791:u64[])  [unwired: 1 in]
                    }
                    n2224 = Transpose 2D Array(2D array=w3781) -> (transposed array=w3786:u64[][])
                    n2225 = Divide(x=w3784, y=w3783) -> (x/y=w3785:dbl)
                    n2226 = Reshape Array(w3786, w3785) -> (w3782:u64[])
                  }
                }
                n2227 = case shown="True" w3710 {
                  tunnel: w3770 -> [w3802 w3814]
                  tunnel: [w3802 w3806] -> w3766
                  tunnel: "Save ave N" -> [_ w3807]
                  tunnel: w3761 -> [_ w3805]
                  frame False {
                    # "don't downsample data for trap calibration"
                  }
                  frame True {
                    n2228 = Array Size(array=w3814) -> (size(s)=w3808:i32)
                    n2229 = Array Size(array=w3805) -> (size(s)=w3804:i32)
                    n2230 = Divide(x=w3808, y=w3804) -> (x/y=w3812:dbl)
                    n2231 = Reshape Array(w3814, w3812, w3804) -> (w3813:i16[][])
                    n2232 = Transpose 2D Array(2D array=w3813) -> (transposed array=w3811:i16[][])
                    n2233 = for {
                      tunnel: w3811 -> [w3817] mode=indexing
                      tunnel: [w3816] -> w3803 mode=indexing
                      tunnel: w3807 -> [w3815]
                      workers-P: _ -> [_]
                      n2234 = call "downsample 1D array - I16.vi"("Ave N"=w3815, "Array In"=w3817) -> ("Array Out"=w3816:i16[])  [unwired: 1 out]
                    }
                    n2235 = Transpose 2D Array(2D array=w3803) -> (transposed array=w3810:i16[][])
                    n2236 = Divide(x=w3808, y=w3807) -> (x/y=w3809:dbl)
                    n2237 = Reshape Array(w3810, w3809) -> (w3806:i16[])
                  }
                }
                n2238 = Index Array(array=w3732, index=1) -> (element=w3735:waveform(dbl))
                n2239 = Index Array(array=w3732, index=0) -> (element=w3737:waveform(dbl))
                n2240 = Unbundle By Name(w3735) -> ("Y"=w3739:dbl[])
                n2241 = Unbundle By Name(w3737) -> ("Y"=w3747:dbl[])
                n2242 = case "Write trap pos. data" shown="True" w3713 {
                  tunnel: w3712 -> [_ w3795]
                  tunnel: w3708 -> [_ w3794]
                  frame False {
                  }
                  frame True {
                    n2243 = Write to Binary File(file (use dialog)=w3795, data=w3794, 5:FALSE ("prepend array or string size? (T)"), 9:T30."big-endian, network order" ("byte order (0:big-endian, network order)")) -> ()  [unwired: 1 in, 4 out]
                  }
                }
                n2244 = Write to Binary File(file (use dialog)=w3773, data=w3766, 5:FALSE ("prepend array or string size? (T)"), 9:T30."big-endian, network order" ("byte order (0:big-endian, network order)")) -> ()  [unwired: 1 in, 4 out]
                n2245 = feedback #26(w3739) -> (w3741:dbl[])
                n2246 = Build Array (concatenate)(w3741, w3739) -> (w3740:dbl[])
                n2247 = Select(t=w3739, s=w3715, f=w3740) -> (s? t:f=w3725:dbl[])
                n2248 = feedback-in #26(w3725) -> ()
                n2249 = feedback #27(w3747) -> (w3760:dbl[])
                n2250 = Build Array (concatenate)(w3760, w3747) -> (w3759:dbl[])
                n2251 = Select(t=w3747, s=w3715, f=w3759) -> (s? t:f=w3734:dbl[])
                n2252 = feedback-in #27(w3734) -> ()
                n2253 = Divide(x=w3774, y=w3775) -> (x/y=w3777:dbl)
                n2254 = Multiply(x=w3777, y=100.0) -> (x*y=w3776:dbl)
                n2255 = Build Array(w3734, w3725) -> (→"Saved APD":dbl[][])
                n2256 = Array Size(array=w3734) -> (size(s)=w3752:i32)
                n2257 = Unbundle By Name(w3754) -> ("Y"=w3758:dbl[])
                n2258 = Subtract(x=w3752, y="N pts to average") -> (x-y=w3728:i32)
                n2259 = Multiply(x="N pts to average", y=u16 2) -> (x*y=w3729:u16)
                n2260 = Subtract(x=w3752, y=w3729) -> (x-y=w3727:i32)
                n2261 = feedback #28(w3758) -> (w3757:dbl[])
                n2262 = Build Array (concatenate)(w3757, w3758) -> (w3756:dbl[])
                n2263 = Select(t=w3758, s=w3715, f=w3756) -> (s? t:f=w3755:dbl[])
                "Trap Delta Graph" <- w3755
                n2264 = feedback-in #28(w3755) -> ()
                n2265 = Array Subset(array=w3734, index=w3728, length="N pts to average") -> (w3751:dbl[])
                n2266 = Array Subset(array=w3734, index=w3727, length="N pts to average") -> (w3750:dbl[])
                n2267 = Array Subset(array=w3725, index=w3728, length="N pts to average") -> (w3731:dbl[])
                n2268 = Array Subset(array=w3725, index=w3727, length="N pts to average") -> (w3730:dbl[])
                n2269 = call-poly <vilib>:"Mean.vi"("X"=w3751) -> ("mean"=w3749:dbl)  [unwired: 1 out]
                n2270 = call-poly <vilib>:"Mean.vi"("X"=w3731) -> ("mean"=w3724:dbl)  [unwired: 1 out]
                n2271 = call-poly <vilib>:"Mean.vi"("X"=w3750) -> ("mean"=w3748:dbl)  [unwired: 1 out]
                n2272 = call-poly <vilib>:"Mean.vi"("X"=w3730) -> ("mean"=w3723:dbl)  [unwired: 1 out]
                n2273 = Subtract(x=w3724, y=w3723) -> (x-y=w3714:dbl)
                "Delta Fl. 2" <- w3714
                n2274 = Subtract(x=w3749, y=w3748) -> (x-y=w3746:dbl)
                "Delta Fl. 1" <- w3746
                n2275 = Initialize Array(w3746, 1 ("dimension size")) -> (w3743:dbl[])
                n2276 = Initialize Array(w3714, 1 ("dimension size")) -> (w3720:dbl[])
                n2277 = feedback #29(w3743) -> (w3744:dbl[])
                n2278 = Build Array (concatenate)(w3744, w3743) -> (w3742:dbl[])
                n2279 = feedback #30(w3720) -> (w3721:dbl[])
                n2280 = Build Array (concatenate)(w3721, w3720) -> (w3719:dbl[])
                n2281 = Select(t=w3743, s=w3715, f=w3742) -> (s? t:f=w3718:dbl[])
                n2282 = feedback-in #29(w3718) -> ()
                n2283 = Select(t=w3720, s=w3715, f=w3719) -> (s? t:f=w3717:dbl[])
                n2284 = feedback-in #30(w3717) -> ()
                n2285 = Build Array(w3718, w3717) -> (→"Save APD Deriv":dbl[][])
              }
            }
            "Progress" <- w3691
            "Progress 2" <- w3691
          }
        }
      }
    }
    n2286 = Bundle By Name(cluster=w2341, "Green FB Ch 0"=w2340, "Green FB Ch 1"=w2339) -> (w2323:T49)
    "Green FB Signals (V)" <- w2323
    n2287 = Unbundle By Name(w2323) -> ("Green FB Ch 2"=→"Green FB Plot":dbl)
    n2288 = local read "wait to reset values"() -> (w2409:bool)
    n2289 = Not(x=w2406) -> (.not. x?=w2410:bool)
    n2290 = And(x=w2410, y=w2409) -> (x .and. y?=w2411:bool)
    n2291 = case "Part of MCL raster scanning: returns to initial positions after scan done" shown="False" w2411 {
      tunnel: w2414 -> [w3243 w3250]
      tunnel: [w3243 w3249] -> w2413
      tunnel: w2408 -> [w3242 w3248]
      tunnel: [w3242 w3247] -> w2407
      frame False {
      }
      frame True {
        w3258 = 10.0 ("y")
        w3257 = 32767.0 ("y")
        # "to return scan values\nafter a synchronous \nAOM scan"
        n2292 = local read "AO2"() -> (w3251:dbl)
        n2293 = local read "AO1"() -> (w3252:dbl)
        n2294 = local write "wait to reset values"(FALSE ("wait to reset values")) -> ()
        n2295 = Multiply(x=w3252, y=w3257) -> (x*y=w3254:dbl)
        n2296 = Multiply(x=w3251, y=w3257) -> (x*y=w3256:dbl)
        n2297 = Divide(x=w3254, y=w3258) -> (x/y=w3253:dbl)
        n2298 = Divide(x=w3256, y=w3258) -> (x/y=w3255:dbl)
        n2299 = To Word Integer(number=w3253) -> (16bit integer=w3259:i16)
        n2300 = To Word Integer(number=w3255) -> (16bit integer=w3260:i16)
        n2301 = local read "Total Counts (ticks)"() -> (w3244:u32)
        n2302 = xnode "Read/Write Control"("FPGA VI Reference In"=w3250, "error in"=w3248, "AO1"=w3259, "AO2"=w3260, "MCL count"=w3244) -> ("FPGA VI Reference Out"=w3249:T20, "error out"=w3247:errorcluster)
        n2303 = local read "Scan Range (V)\n(of steps)"() -> (w3245:dbl)
        n2304 = property on="Scan Range (V)\n(of steps)" class="DigNum (strict)"("Val(Sgnl)"=w3245) -> ()  [unwired: 2 in, 2 out]
      }
    }
    n2305 = node-c288() -> ()  [unwired: 2 out]
  }
  n2306 = node-c288(3 ("Processor")) -> (w94:T25)  [unwired: 3 out]
  n2307 = timed-loop "Oscillate AOD (debugging)" {
    tunnel: w44 -> [w3819]
    tunnel: [w3818] -> w56
    timing: w94 -> [_]
    timing-out: [_] -> w93
    stop <- w3818 stop-if-true
    n2308 = node-c288() -> ()  [unwired: 2 out]
    n2309 = event shown="[0] \"Oscillate Set 2\", \"Fish for Tether\": Value Change" {
      selector: _ -> [_ _ _]
      dyn-events: _ -> [_ _ _]
      timeout: _ -> [_ _ _]
      tunnel: w3819 -> [w3826 _ _]
      tunnel: [FALSE ("Stop All") _ w4094] -> w3818
      event "Oscillate Set 2", "Fish for Tether": Value Change {
        n2310 = event-data() -> ()  [unwired: 6 out]
        n2311 = local read "Oscillate Set 2"() -> (w3825:bool)
        n2312 = Or(x=w3825, y="Fish for Tether") -> (x .or. y?=w3823:bool)
        n2313 = case shown="True" w3823 {
          tunnel: w3826 -> [_ w3829]
          tunnel: "Fish for Tether" -> [_ w3828]
          frame False {
          }
          frame True {
            n2314 = case shown="True" w3828 {
              frame False {
              }
